vi "VII Write Bytes.vi"(4 "Len":u16, 6 "SubAddr":i32, 7 "SlaveAddr":u16, 9 "I2CIndex":i32, 10 "DevIndex":i32, 11 "DevType":i32) -> (3 "function return":i32)   [LabVIEW 2012, in "ControlI2C.lvlib"]
doc: "int __stdcall VII_WriteBytes(int DevType,int DevIndex,int I2CIndex,unsigned short SlaveAddr,int SubAddr,unsigned char *pWriteData,unsigned short Len);"
uses:
  ControlI2C.lvlib
  Ginkgo_Driver.dll
panel:
  in  "pWriteData":u8[](array[numeric])=array[10240 elements]
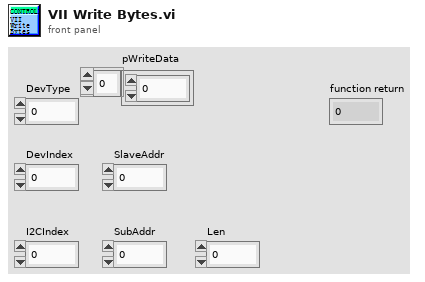
[diagram p1: front panel]
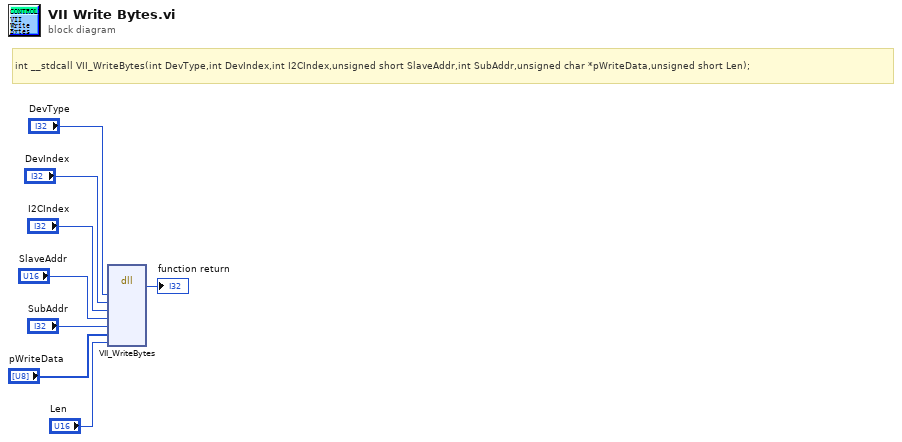
[diagram p0: block diagram]
diagram:
  # "int __stdcall VII_WriteBytes(int DevType,int DevIndex,int I2CIndex,unsigned short SlaveAddr,int SubAddr,unsigned char *pWriteData,unsigned short Len);"
  n1 = dll-call lib="E:/Project/vt_ginkgo/truck/Ginkgo Driver/vs2010/Ginkgo_USB-I2C&SPI&CAN_API_v2.0.3.5/lib/labview_32bit/ControlI2C/Ginkgo_Driver.*" fn="VII_WriteBytes"("DevType"="DevType", "DevIndex"="DevIndex", "I2CIndex"="I2CIndex", "SlaveAddr"="SlaveAddr", "SubAddr"="SubAddr", "pWriteData"="pWriteData", "Len"="Len") -> ("return type"=→"function return":i32)  [unwired: 10 in, 2 out]
